vi "(SubVI) Find initial centeringdata center.vi"(4 "QPD array (V)":dbl[](array[numeric]), 5 "Stage array (um)":dbl[](array[numeric])) -> (0 "Initial guess QPD center (yr) (V)":dbl, 2 "Initial guess stage center (cr) (um)":dbl)   [LabVIEW 2014]
uses:
  <vilib>/Analysis/baseanly.llb/Mean (DBL).vi
  <vilib>/Analysis/NI_AALBase.lvlib
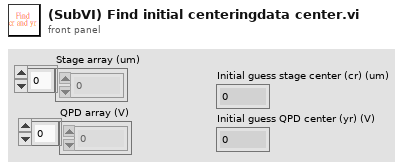
[diagram p1: front panel]
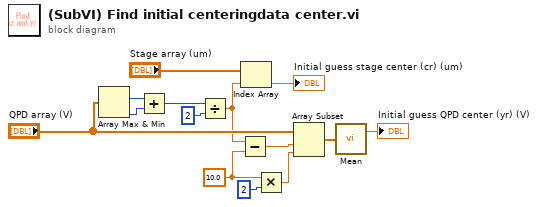
[diagram p0: block diagram]
diagram:
  w4 = 10.0 ("y")
  n1 = Array Max & Min(array="QPD array (V)") -> (max index (indices)=w13:i32, min index (indices)=w12:i32)  [unwired: 2 out]
  n2 = Add(x=w13, y=w12) -> (x+y=w11:i32)
  n3 = Divide(x=w11, y=2) -> (x/y=w7:dbl)
  n4 = Subtract(x=w7, y=w4) -> (x-y=w6:dbl)
  n5 = Index Array(array="Stage array (um)", index=w7) -> (element=→"Initial guess stage center (cr) (um)":dbl)
  n6 = Multiply(x=w4, y=2) -> (x*y=w3:dbl)
  n7 = Array Subset(array="QPD array (V)", index=w6, length=w3) -> (w2:dbl[])
  n8 = call-poly <vilib>:"Mean.vi"("X"=w2) -> ("mean"=→"Initial guess QPD center (yr) (V)":dbl)  [unwired: 1 out]
